vi "update_features.vi"(6 "payload":string, 8 "Path to creds.json file":path=path "/Users/milandahal/Documents/GitHub/Onshape/python/creds.json", 9 "wid":string, 10 "did":string, 11 "eid":string) -> (0 "Output Body":string, 3 "Output headers":string)   [LabVIEW 2019]
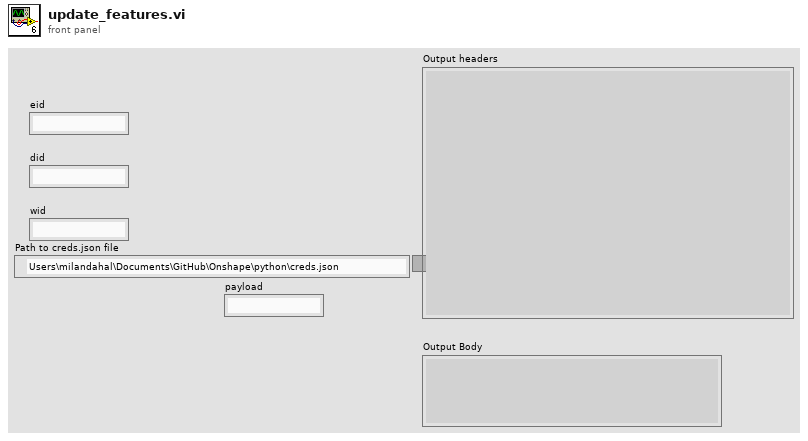
[diagram p1: front panel]
types:
  T1 = cluster{"Date":string, "On-Nonce":string, "ctype":string, "path":string, "method":string, "Authorization":string, "Accept":string, "User-Agent":string, "Content-Type":string, "secret_key":string, "access_key":string, "stack":string, "payload":string}
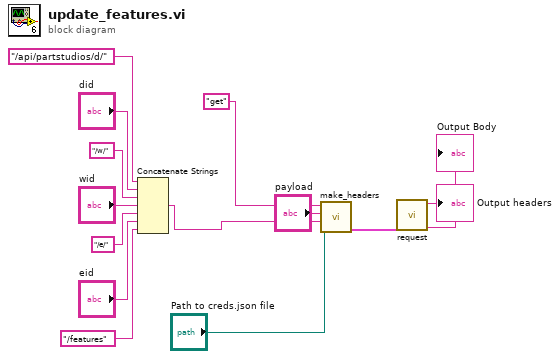
[diagram p0: block diagram]
diagram:
  n1 = Concatenate Strings("/api/partstudios/d/" ("payload"), "did", "/w/" ("string"), "wid", "/e/" ("string"), "eid", "/features" ("string")) -> (w6:string)
  n2 = call "make_headers.vi"("Method"="get", "payload"="payload", "path"=w6, "Path to creds.json file"="Path to creds.json file") -> ("output cluster"=w4:T1)  [unwired: 5 in, 1 out]
  n3 = call "request.vi"("input cluster"=w4) -> ("Output headers"=→"Output headers":string, "Output Body"=→"Output Body":string)  [unwired: 7 in]
